vi "Register for Listen Events.vi"(8 "error in (no error)":errorcluster, 11 "CIFCorePlugin in":refnum<class "CIFCorePlugin.lvclass">) -> (0 "error out":errorcluster, 3 "Listen Event refnum":refnum<event-registration>)   [LabVIEW 2021, in "CIFCorePlugin.lvclass"]
uses:
  CIFCorePlugin.lvclass
  CIFCorePlugin.lvclass/CIFCorePlugin.ctl
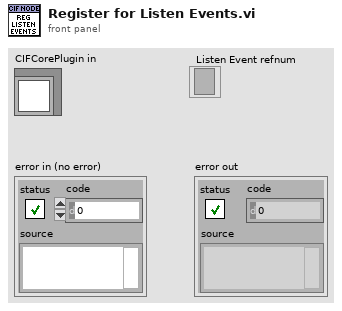
[diagram p1: front panel]
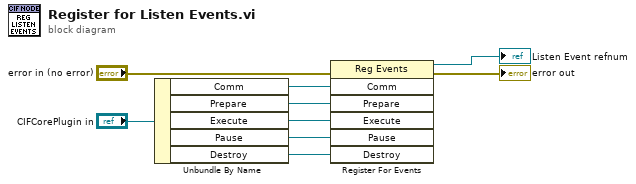
[diagram p0: block diagram]
diagram:
  n1 = Unbundle By Name("CIFCorePlugin in") -> ("Comm"=w8:refnum<user-event>, "Prepare"=w7:refnum<user-event>, "Execute"=w6:refnum<user-event>, "Pause"=w5:refnum<user-event>, "Destroy"=w4:refnum<user-event>)
  n2 = register-events(error in="error in (no error)", w8, w7, w6, w5, w4) -> (reference out=→"Listen Event refnum":refnum<event-registration>, error out=→"error out":errorcluster)  [unwired: 1 in]
